vi "SQL.Statistic_TestItem.vi"(7 "最大查询天数":u32, 9 "索引测试值":i32, 10 "Date":string, 11 "Folder Path":path caption="文件夹路径") -> (0 "密度图":cluster{cluster{dbl, i32}[]}[](graph), 1 "分布图":cluster{cluster{i32, dbl}[]}[](graph), 3 "统计数据输出":T1 {"均值" format="%0.2f"; "方差" format="%0.2f"; "最大值" format="%0.2f"})   [LabVIEW 2012, in "Lib_UEL.ATE.lvlib" / "Lib_SQL.lvlib"]
uses:
  Lib_SQL.lvlib
  <vilib>/Analysis/NI_AALBase.lvlib
  <vilib>/Analysis/NI_AALPro.lvlib
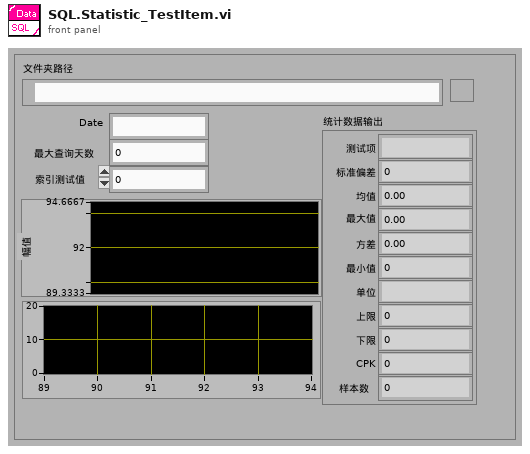
[diagram p1: front panel]
types:
  T1 = cluster{"测试项":string, "单位":string, "上限":dbl, "下限":dbl, "均值":dbl, "最大值":dbl, "最小值":dbl, "方差":dbl, "标准偏差":dbl, "CPK":dbl, "样本数":i32}
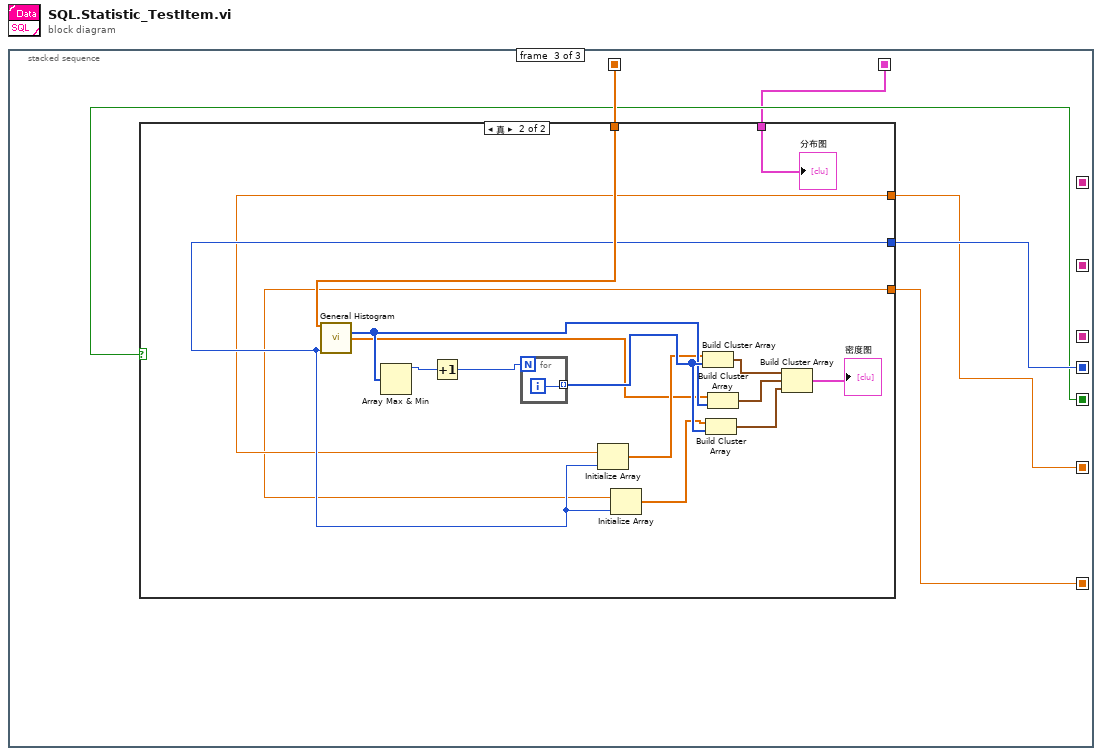
[diagram p0: block diagram]
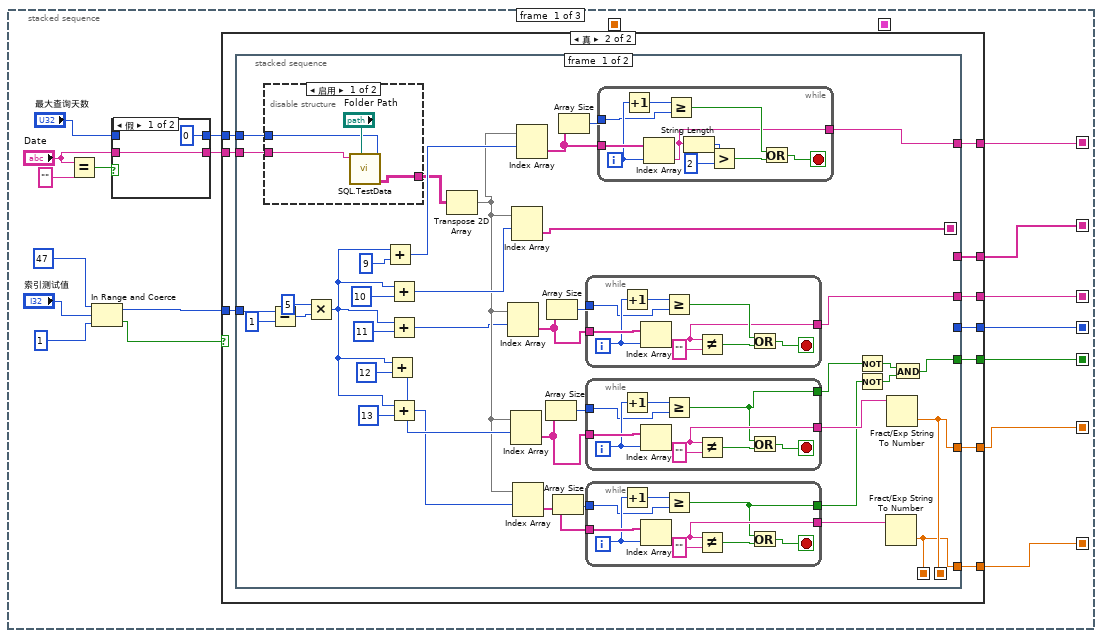
[diagram p2: hidden frame]
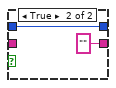
[diagram p3: hidden frame]
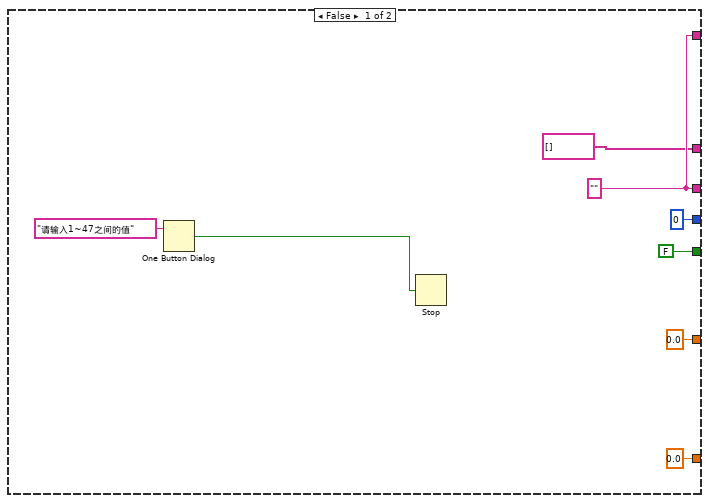
[diagram p4: hidden frame]
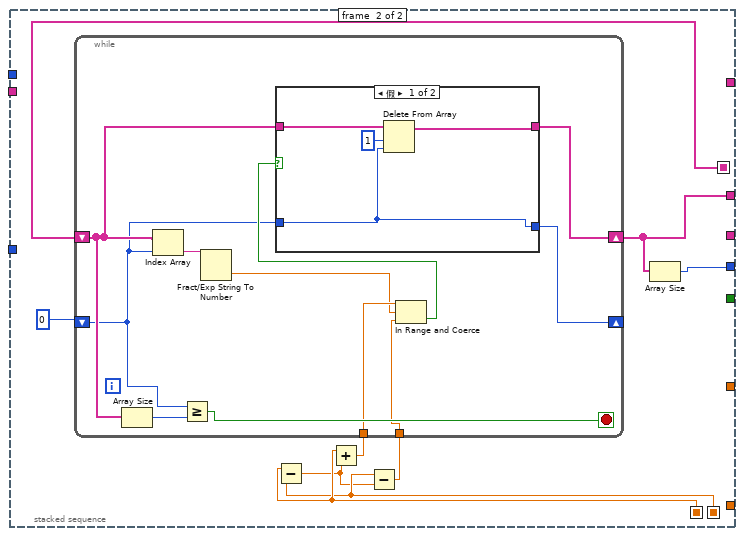
[diagram p6: hidden frame]
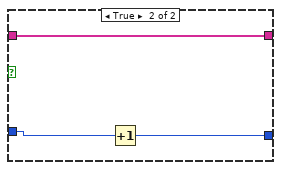
[diagram p7: hidden frame]
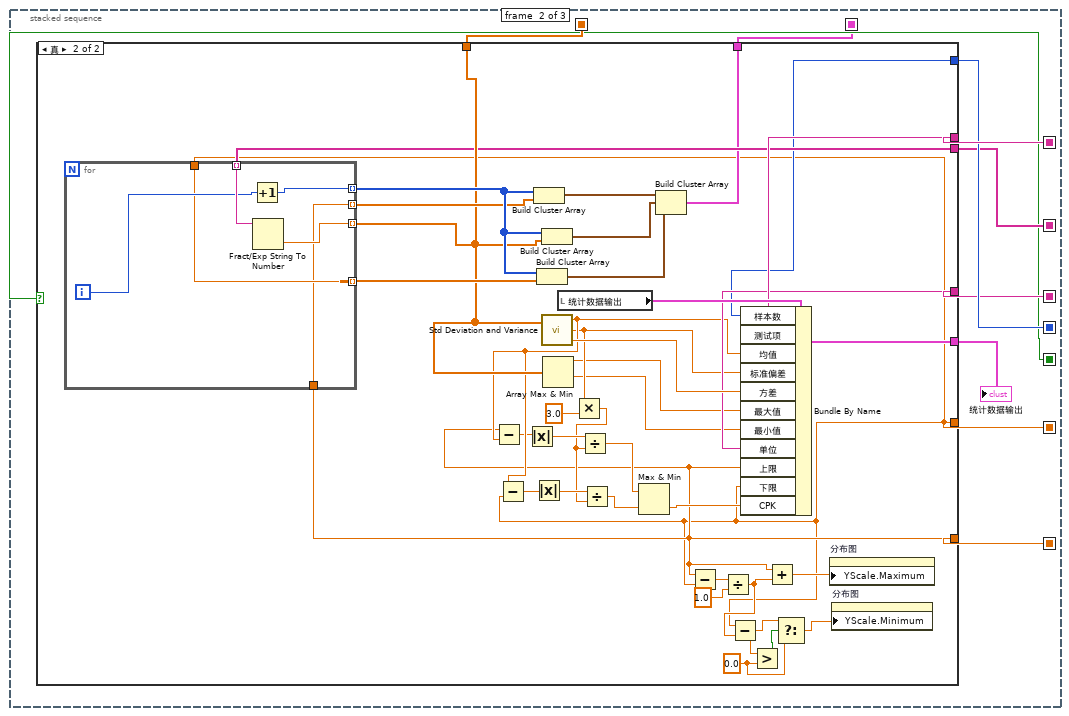
[diagram p8: hidden frame]
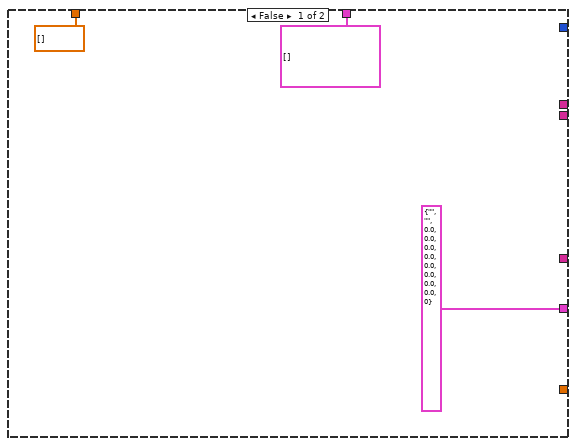
[diagram p9: hidden frame]
diagram:
  n1 = stacked-sequence {
    seq-local: [_ w157 _] -> [_ _ w210]
    seq-local: [w13 _ _] -> [_ w152 _]
    seq-local: [w12 _ _] -> [_ w155 _]
    seq-local: [w11 _ _] -> [_ w150 w208]
    seq-local: [w10 _ _] -> [_ w151 w207]
    seq-local: [w9 _ _] -> [_ w153 _]
    seq-local: [w8 _ _] -> [_ w154 w209]
    seq-local: [w7 _ _] -> [_ w149 w206]
    seq-local: [_ w148 _] -> [_ _ w205]
    frame #0 {
      n2 = Equal?(x="Date", y="") -> (x = y?=w5:bool)
      n3 = In Range and Coerce(upper limit=47 ("上限"), x="索引测试值", lower limit=1 ("下限")) -> (coerced(x)=w14:i32, In Range?=w16:bool)
      n4 = case shown="假" w5 {
        tunnel: [w20 "" ("Date")] -> w4
        tunnel: "Date" -> [w20 _]
        tunnel: "最大查询天数" -> [_ w22]
        tunnel: [u32 0 ("最大查询天数") w22] -> w1
        frame False {
        }
        frame True {
        }
      }
      n5 = case shown="真" w16 {
        tunnel: w14 -> [_ w40]
        tunnel: [w28 w39] -> w13
        tunnel: [w28 w38] -> w12
        tunnel: [0.0 w37] -> w11
        tunnel: [0.0 w36] -> w10
        tunnel: [string[] [] w35] -> w9
        tunnel: [0 w34] -> w8
        tunnel: [FALSE w33] -> w7
        tunnel: w4 -> [_ w32]
        tunnel: w1 -> [_ w31]
        frame False {
          w28 = ""
          n6 = One Button Dialog(message="请输入1~47之间的值" ("消息")) -> (true=w29:bool)  [unwired: 1 in]
          n7 = Stop(stop? (T)=w29) -> ()
        }
        frame True {
          n8 = stacked-sequence {
            seq-local: [w50 _] -> [_ w127]
            seq-local: [w49 _] -> [_ w128]
            seq-local: [w48 _] -> [_ w129]
            tunnel: w40 -> [w68 _]
            tunnel: [w56 _] -> w39
            tunnel: [w53 _] -> w38
            tunnel: [w50 _] -> w37
            tunnel: [w49 _] -> w36
            tunnel: [_ w123] -> w35
            tunnel: [_ w122] -> w34
            tunnel: [w47 _] -> w33
            tunnel: w32 -> [w42 _]
            tunnel: w31 -> [w41 _]
            frame #0 {
              n9 = disable-structure shown="启用" {
                disable-tunnel: [w120 _] -> w70
                disable-tunnel: w42 -> [w118 _]
                disable-tunnel: w41 -> [w117 _]
                frame Enabled {
                  n10 = call "SQL.TestData.vi"("最大查询天数"=w117, "Folder Path"="Folder Path", "Date"=w118) -> ("SQL Results"=w120:string[][])  [unwired: 6 in, 2 out]
                }
                frame Disabled {
                }
              }
              n11 = Subtract(x=w68, y=1) -> (x-y=w78:i32)
              n12 = Multiply(x=5, y=w78) -> (x*y=w66:i32)
              n13 = Add(x=w66, y=9 ("x")) -> (x+y=w76:i32)
              n14 = Add(x=w66, y=u32 12) -> (x+y=w72:u32)
              n15 = Add(x=w66, y=10 ("x")) -> (x+y=w75:i32)
              n16 = Add(x=w66, y=11 ("x")) -> (x+y=w63:i32)
              n17 = Add(x=w66, y=u32 13) -> (x+y=w71:u32)
              n18 = Transpose 2D Array(2D array=w70) -> (transposed array=w64:string[][])
              n19 = Index Array(array=w64, index (row)=w63) -> (element=w58:string[])  [unwired: 1 in]
              n20 = Index Array(array=w64, index (row)=w72) -> (element=w59:string[])  [unwired: 1 in]
              n21 = Index Array(array=w64, index (row)=w75) -> (element=w48:string[])  [unwired: 1 in]
              n22 = Index Array(array=w64, index (row)=w71) -> (element=w62:string[])  [unwired: 1 in]
              n23 = Index Array(array=w64, index (row)=w76) -> (element=w54:string[])  [unwired: 1 in]
              n24 = Array Size(array=w59) -> (size(s)=w60:i32)
              n25 = Array Size(array=w58) -> (size(s)=w57:i32)
              n26 = Array Size(array=w62) -> (size(s)=w61:i32)
              n27 = Array Size(array=w54) -> (size(s)=w55:i32)
              n28 = while {
                tunnel: w58 -> [w98]
                tunnel: w57 -> [w94]
                tunnel: [w90] -> w56
                i -> [w95]
                stop <- w93 stop-if-true
                n29 = Increment(x=w95) -> (x+1=w96:i32)
                n30 = Index Array(array=w98, index=w95) -> (element=w90:string)
                n31 = Greater Or Equal?(x=w96, y=w94) -> (x >= y?=w91:bool)
                n32 = Not Equal?(x=w90, y="") -> (x != y?=w92:bool)
                n33 = Or(x=w91, y=w92) -> (x .or. y?=w93:bool)
              }
              n34 = while {
                tunnel: w59 -> [w107]
                tunnel: w60 -> [w103]
                tunnel: [w100] -> w52
                tunnel: [w99] -> w46
                i -> [w104]
                stop <- w102 stop-if-true
                n35 = Increment(x=w104) -> (x+1=w105:i32)
                n36 = Index Array(array=w107, index=w104) -> (element=w100:string)
                n37 = Greater Or Equal?(x=w105, y=w103) -> (x >= y?=w99:bool)
                n38 = Not Equal?(x=w100, y="") -> (x != y?=w101:bool)
                n39 = Or(x=w99, y=w101) -> (x .or. y?=w102:bool)
              }
              n40 = while {
                tunnel: w62 -> [w116]
                tunnel: w61 -> [w112]
                tunnel: [w109] -> w51
                tunnel: [w108] -> w45
                i -> [w113]
                stop <- w111 stop-if-true
                n41 = Increment(x=w113) -> (x+1=w114:i32)
                n42 = Index Array(array=w116, index=w113) -> (element=w109:string)
                n43 = Greater Or Equal?(x=w114, y=w112) -> (x >= y?=w108:bool)
                n44 = Not Equal?(x=w109, y="") -> (x != y?=w110:bool)
                n45 = Or(x=w108, y=w110) -> (x .or. y?=w111:bool)
              }
              n46 = while {
                tunnel: w54 -> [w89]
                tunnel: w55 -> [w86]
                tunnel: [w80] -> w53
                i -> [w87]
                stop <- w85 stop-if-true
                n47 = Increment(x=w87) -> (x+1=w88:i32)
                n48 = Index Array(array=w89, index=w87) -> (element=w80:string)
                n49 = Greater Or Equal?(x=w88, y=w86) -> (x >= y?=w83:bool)
                n50 = String Length(string=w80) -> (length=w82:i32)
                n51 = Greater?(x=w82, y=2) -> (0:w84:bool)
                n52 = Or(x=w83, y=w84) -> (x .or. y?=w85:bool)
              }
              n53 = Not(x=w46) -> (.not. x?=w43:bool)
              n54 = Not(x=w45) -> (.not. x?=w44:bool)
              n55 = Fract/Exp String To Number(string=w51) -> (number=w49:dbl)  [unwired: 3 in, 1 out]
              n56 = Fract/Exp String To Number(string=w52) -> (number=w50:dbl)  [unwired: 3 in, 1 out]
              n57 = And(x=w43, y=w44) -> (x .and. y?=w47:bool)
            }
            frame #1 {
              n58 = Subtract(x=w128, y=w127) -> (x-y=w126:dbl)
              n59 = Add(x=w128, y=w126) -> (x+y=w125:dbl)
              n60 = Subtract(x=w127, y=w126) -> (x-y=w124:dbl)
              n61 = while {
                shift-right: [w133] -> w123
                shift-left: w129 -> [w132]
                tunnel: w125 -> [w137]
                tunnel: w124 -> [w136]
                shift-right: [w130] -> _
                shift-left: 0 ("下限") -> [w131]
                stop <- w139 stop-if-true
                n62 = Array Size(array=w132) -> (size(s)=w140:i32)
                n63 = Index Array(array=w132, index=w131) -> (element=w138:string)
                n64 = Greater Or Equal?(x=w131, y=w140) -> (x >= y?=w139:bool)
                n65 = Fract/Exp String To Number(string=w138) -> (number=w135:dbl)  [unwired: 3 in, 1 out]
                n66 = In Range and Coerce(upper limit=w137, x=w135, lower limit=w136) -> (In Range?=w134:bool)  [unwired: 1 out]
                n67 = case shown="假" w134 {
                  tunnel: [w142 w147] -> w133
                  tunnel: w132 -> [w144 w147]
                  tunnel: w131 -> [w141 w146]
                  tunnel: [w141 w145] -> w130
                  frame False {
                    n68 = Delete From Array(array=w144, length=1 ("长度"), index=w141) -> (array with subset deleted=w142:string[])  [unwired: 1 out]
                  }
                  frame True {
                    n69 = Increment(x=w146) -> (x+1=w145:i32)
                  }
                }
              }
              n70 = Array Size(array=w123) -> (size(s)=w122:i32)
            }
          }
        }
      }
    }
    frame #1 {
      n71 = case shown="真" w149 {
        tunnel: [dbl[] [] w193] -> w157
        tunnel: [T1 {"测试项"="", "单位"="", "上限"=0.0, "下限"=0.0, "均值"=0.0, "最大值"=0.0, "最小值"=0.0, "方差"=0.0, "标准偏差"=0.0, "CPK"=0.0, "样本数"=0} ("统计数据输出") w191] -> w156
        tunnel: w155 -> [_ w189]
        tunnel: w154 -> [_ w175]
        tunnel: w153 -> [_ w188]
        tunnel: w152 -> [_ w187]
        tunnel: w151 -> [_ w162]
        tunnel: w150 -> [_ w161]
        tunnel: [cluster{cluster{i32, dbl}[]}[] [] w173] -> w148
        frame False {
        }
        frame True {
          w165 = 0.0 ("y")
          n72 = for {
            tunnel: [w199] -> w194 mode=indexing
            tunnel: [w204] -> w196 mode=indexing
            tunnel: [w200] -> w195 mode=indexing
            tunnel: [w202] -> w193 mode=indexing
            tunnel: w188 -> [w203] mode=indexing
            tunnel: w161 -> [w200]
            tunnel: w162 -> [w199]
            i -> [w201]
            n73 = Increment(x=w201) -> (x+1=w204:i32)
            n74 = Fract/Exp String To Number(string=w203) -> (number=w202:dbl)  [unwired: 3 in, 1 out]
          }
          n75 = Build Cluster Array(w196, w194) -> (w198:cluster{i32, dbl}[])
          n76 = Build Cluster Array(w196, w195) -> (w197:cluster{i32, dbl}[])
          n77 = Build Cluster Array(w196, w193) -> (w174:cluster{i32, dbl}[])
          n78 = call <vilib>:"Std Deviation and Variance.vi"("X"=w193) -> ("mean"=w186:dbl, "standard deviation"=w181:dbl, "variance"=w190:dbl)  [unwired: 1 in]
          n79 = Subtract(x=w162, y=w186) -> (x-y=w185:dbl)
          n80 = Subtract(x=w186, y=w161) -> (x-y=w184:dbl)
          n81 = Absolute Value(x=w185) -> (abs(x)=w182:dbl)
          n82 = Absolute Value(x=w184) -> (abs(x)=w183:dbl)
          n83 = Array Max & Min(array=w193) -> (max value=w171:dbl, min value=w168:dbl)  [unwired: 2 out]
          n84 = local read "统计数据输出"() -> (w192:T1)
          n85 = Multiply(x=w181, y=3.0) -> (x*y=w179:dbl)
          n86 = Divide(x=w182, y=w179) -> (x/y=w178:dbl)
          n87 = Divide(x=w183, y=w179) -> (x/y=w177:dbl)
          n88 = Max & Min(x=w178, y=w177) -> (min(x,y)=w176:dbl)  [unwired: 1 out]
          n89 = Build Cluster Array(w198, w174, w197) -> (w173:cluster{cluster{i32, dbl}[]}[])
          n90 = Subtract(x=w162, y=w161) -> (x-y=w172:dbl)
          n91 = Divide(x=w172, y=1.0) -> (x/y=w167:dbl)
          n92 = Subtract(x=w161, y=w167) -> (x-y=w166:dbl)
          n93 = Bundle By Name(cluster=w192, "样本数"=w175, "测试项"=w189, "均值"=w186, "标准偏差"=w181, "方差"=w190, "最大值"=w171, "最小值"=w168, "单位"=w187, "上限"=w162, "下限"=w161, "CPK"=w176) -> (w191:T1)
          n94 = Greater?(x=w166, y=w165) -> (0:w164:bool)
          n95 = Add(x=w162, y=w167) -> (x+y=w170:dbl)
          n96 = Select(t=w166, s=w164, f=w165) -> (s? t:f=w163:dbl)
          n97 = property on="分布图" class="XYGraph (严格)"("YScale.Maximum"=w170) -> ()  [unwired: 2 in, 2 out]
          n98 = property on="分布图" class="XYGraph (严格)"("YScale.Minimum"=w163) -> ()  [unwired: 2 in, 2 out]
        }
      }
      "统计数据输出" <- w156
    }
    frame #2 {
      n99 = case shown="真" w206 {
        tunnel: w210 -> [_ w216]
        tunnel: w209 -> [_ w214]
        tunnel: w208 -> [_ w213]
        tunnel: w207 -> [_ w212]
        tunnel: w205 -> [_ w211]
        frame False {
        }
        frame True {
          n100 = call <vilib>:"General Histogram.vi"("X"=w216, "# bins"=w214) -> ("Histogram"=w222:i32[], "Axis"=w219:dbl[])  [unwired: 9 in, 3 out]
          n101 = Array Max & Min(array=w222) -> (max value=w223:i32)  [unwired: 3 out]
          n102 = Increment(x=w223) -> (x+1=w224:i32)
          n103 = for {
            N: w224 -> [_]
            tunnel: [w227] -> w226 mode=indexing
            i -> [w227]
          }
          n104 = Initialize Array(w213, w214) -> (w220:dbl[])
          n105 = Initialize Array(w212, w214) -> (w225:dbl[])
          n106 = Build Cluster Array(w220, w226) -> (w218:cluster{dbl, i32}[])
          n107 = Build Cluster Array(w225, w226) -> (w221:cluster{dbl, i32}[])
          n108 = Build Cluster Array(w219, w222) -> (w215:cluster{dbl, i32}[])
          n109 = Build Cluster Array(w218, w215, w221) -> (→"密度图":cluster{cluster{dbl, i32}[]}[])
          "分布图" <- w211
        }
      }
    }
  }
